vi "Exit Test.vi"(8 "error in":errorcluster, 10 "data":variant) -> (0 "error out":errorcluster)   [LabVIEW 2018, in "LED Control Module.lvlib"]
uses:
  LED Control Module.lvlib
  Private Controls/Module Data Cluster.ctl
  Private Controls/Module Action.ctl
  Private Controls/Queue FG Action.ctl
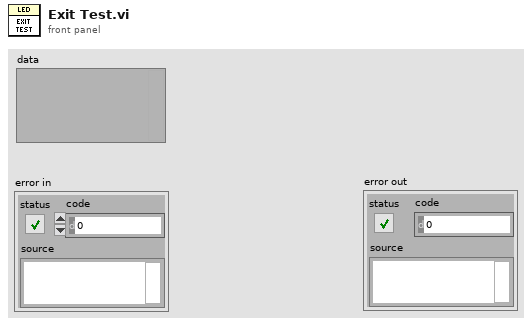
[diagram p1: front panel]
types:
  T1 = typedef "LED Control Module.lvlib/Queue FG Action.ctl" = enum16{"Release", "Get", "Set"}
  T2 = typedef "LED Control Module.lvlib/Module Data Cluster.ctl" = cluster{"Variant":variant, "action":T3}
  T3 = typedef "LED Control Module.lvlib/Module Action.ctl" = enum16{"init", "start", "Current", "Spectrum", "WriteResult", "---WIP---", "clear", "error", "close", "exit"}
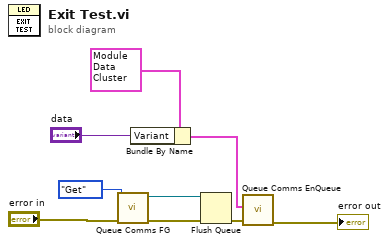
[diagram p0: block diagram]
diagram:
  n1 = call "Queue Comms FG.vi"("error in"="error in", "Action"=Queue_FG_Action."Get") -> ("error out"=w4:errorcluster, "queue out"=w2:refnum<queue>)  [unwired: 8 in]
  n2 = Bundle By Name(cluster=T2 {"Variant"=variant, "action"=enum."exit"} ("Module Data Cluster"), "Variant"="data") -> (w1:T2)
  n3 = Flush Queue(queue=w2, error in (no error)=w4) -> (error out=w6:errorcluster)  [unwired: 2 out]
  n4 = call "Queue Comms EnQueue.vi"("error in"=w6, "Module Data Cluster"=w1) -> ("error out"=→"error out":errorcluster)  [unwired: 9 in]
